vi "Write Coords.vi"(6 "Coordinates":T1, 11 "Populate Menu Msg in":refnum<class "Populate Menu Msg.lvclass">) -> (3 "Populate Menu Msg out":refnum<class "Populate Menu Msg.lvclass">)   [LabVIEW 2017, in "Populate Menu Msg.lvclass"]
uses:
  <vilib>/gpm_packages/@cs/Test-executive-builder/Source/Test Executive Builder View/Test Executive Builder View Messages/Populate Menu Msg/Populate Menu Msg.lvclass
  <vilib>/Utility/miscctls.llb/LVPoint32TypeDef.ctl
  <vilib>/gpm_packages/@cs/Test-executive-builder/Source/Test Executive Builder View/Test Executive Builder View Messages/Populate Menu Msg/Populate Menu Msg.lvclass/Populate Menu Msg.ctl
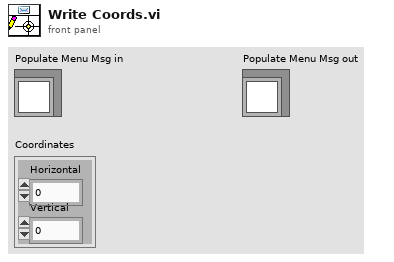
[diagram p1: front panel]
types:
  T1 = typedef "LVPoint32TypeDef.ctl" = cluster{"Horizontal":i32, "Vertical":i32}
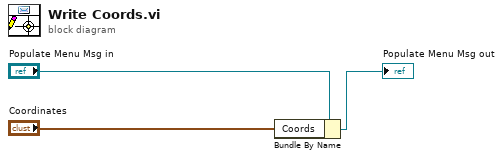
[diagram p0: block diagram]
diagram:
  n1 = Bundle By Name(cluster="Populate Menu Msg in", "Coords"="Coordinates") -> (→"Populate Menu Msg out":refnum<class "Populate Menu Msg.lvclass">)
